vi "Piezo test.vi"() -> ()   [LabVIEW 2017]
panel:
  out "error out":errorcluster
  in  "stop":bool
  in  "Z":dbl
  in  "Y":dbl
  in  "X":dbl
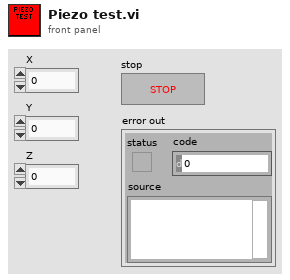
[diagram p1: front panel]
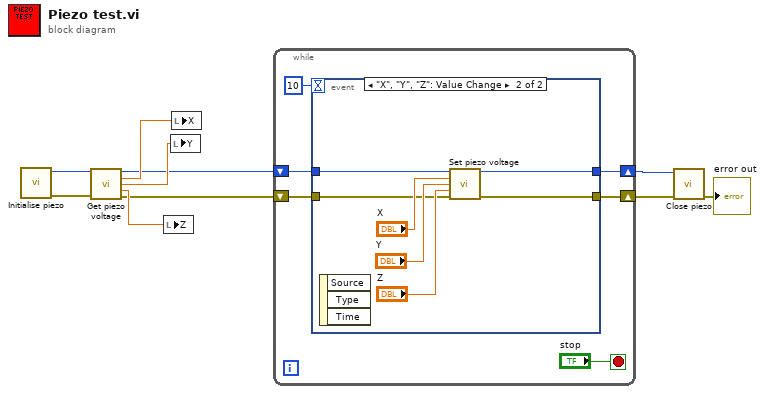
[diagram p0: block diagram]
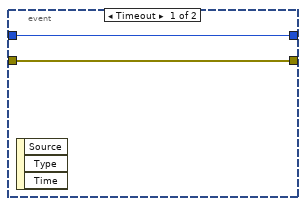
[diagram p2: hidden frame]
diagram:
  n1 = call "Initialise piezo.vi"() -> ("Piezo error out"=w6:errorcluster, "Piezo handle"=w7:i32)  [unwired: 10 in]
  n2 = call "Get piezo voltage.vi"("Piezo handle"=w7, "Piezo error in"=w6) -> ("Piezo handle out"=w5:i32, "X Voltage"=w8:dbl, "Y Voltage"=w9:dbl, "Z Voltage"=w10:dbl, "Piezo error out"=w4:errorcluster)  [unwired: 9 in]
  n3 = local write "Z"(w10) -> ()
  n4 = local write "Y"(w9) -> ()
  n5 = local write "X"(w8) -> ()
  n6 = while {
    shift-right: [w16] -> w3
    shift-left: w5 -> [w14]
    shift-right: [w15] -> w2
    shift-left: w4 -> [w13]
    stop <- "stop" stop-if-true
    n7 = event shown="[1] \"X\", \"Y\", \"Z\": Value Change" {
      selector: _ -> [_ _]
      dyn-events: _ -> [_ _]
      timeout: 10 -> [_ _]
      tunnel: w14 -> [w18 w19]
      tunnel: [w18 w25] -> w16
      tunnel: [w17 w21] -> w15
      tunnel: w13 -> [w17 w20]
      event Timeout {
        n8 = event-data() -> ()  [unwired: 1 in, 3 out]
      }
      event "X", "Y", "Z": Value Change {
        n9 = event-data() -> ()  [unwired: 1 in, 3 out]
        n10 = call "Set piezo voltage.vi"("Piezo handle"=w19, "X Voltage"="X", "Y Voltage"="Y", "Z Voltage"="Z", "Piezo error in"=w20) -> ("Piezo handle out"=w25:i32, "Piezo error out"=w21:errorcluster)  [unwired: 9 in]
      }
    }
  }
  n11 = call "Close piezo.vi"("Piezo error in"=w2, "Piezo handle"=w3) -> ("error out"=→"error out":errorcluster)  [unwired: 9 in]
